vi "Armed Response.vi"(8 "error in (no error)":errorcluster, 9 "Armed":bool, 10 "Sender":string, 11 "Pulse Controller in":refnum<class "Pulse Controller.lvclass">) -> (0 "error out":errorcluster, 3 "Pulse Controller out":refnum<class "Pulse Controller.lvclass">)   [LabVIEW 2016, in "Pulse Controller.lvclass"]
uses:
  Pulse Controller.lvclass
  C:/github/LabActor/Controllers/Process Controller/Process Controller.lvclass
  C:/Program Files/National Instruments/LabVIEW 2016/vi.lib/ActorFramework/Actor/Actor.lvclass
  Process Controller/Process Controller.lvclass/Process Controller.ctl
  Pulse Controller.lvclass/Pulse Controller.ctl
  <vilib>/ActorFramework/Actor/Actor.lvclass/Actor.ctl
  Monitor-Pulse Messages/Update Armed Msg/Update Armed Msg.lvclass/Update Armed Msg.ctl
  <vilib>/ActorFramework/Message Enqueuer/Message Enqueuer.lvclass/Message Enqueuer.ctl
  Process Controller/Read Active measurements names.vi
  <vilib>/ActorFramework/Message Enqueuer/Enqueue.vi
  Monitor-Pulse Messages/Update Armed Msg/Update Armed Msg.lvclass
  C:/Program Files/National Instruments/LabVIEW 2016/vi.lib/ActorFramework/Message/Message.lvclass
  <vilib>/ActorFramework/Message Priority Queue/Priority Enqueue.vi
  <vilib>/ActorFramework/Actor/Actor.lvclass
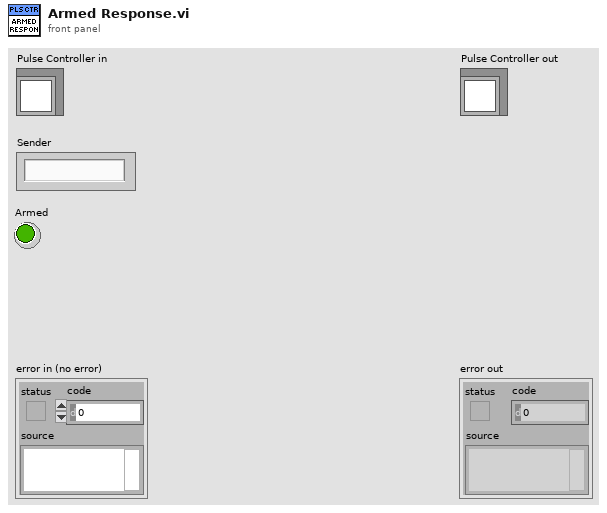
[diagram p1: front panel]
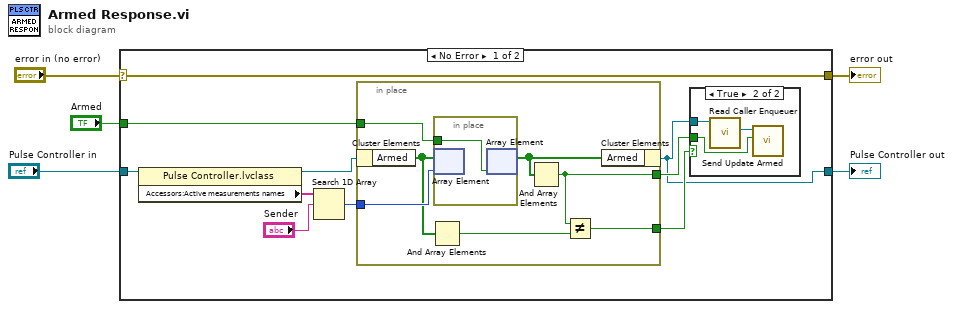
[diagram p0: block diagram]
diagram:
  n1 = case shown="No Error" "error in (no error)" {
    selector: "error in (no error)" -> [w14 w28]
    tunnel: [w14 w28] -> w4
    tunnel: [w6 w27] -> w2
    tunnel: "Pulse Controller in" -> [w15 w27]
    tunnel: "Armed" -> [w10 _]
    frame No Error {
      n2 = property class="Pulse Controller.lvclass"(reference=w15) -> (reference out=w9:refnum<class "Pulse Controller.lvclass">, "Accessors:Active measurements names"=w13:string[])  [unwired: 1 in, 1 out]
      n3 = Search 1D Array(1D array=w13, element="Sender") -> (index of element=w11:i32)  [unwired: 1 in]
      n4 = in-place {
        in-place-border: w11 -> [w25]
        in-place-border: w10 -> [w24]
        in-place-border: [w20] -> w8
        in-place-border: [w19] -> w7
        n5 = in-place-cluster #1(w9) -> ("Armed"=w23:bool[])
        n6 = And Array Elements(Boolean array=w23) -> (logical AND=w21:bool)
        n7 = in-place {
          in-place-border: w24 -> [w26]
          n8 = in-place-array #2(w23, w25) -> ()  [unwired: 1 out]
          n9 = in-place-array #2(w26) -> (w22:bool[])  [unwired: 1 out]
        }
        n10 = And Array Elements(Boolean array=w22) -> (logical AND=w19:bool)
        n11 = Not Equal?(x=w19, y=w21) -> (x != y?=w20:bool)
        n12 = in-place-cluster #1("Armed"=w22) -> (w6:refnum<class "Pulse Controller.lvclass">)
      }
      n13 = case shown="True" w8 {
        tunnel: w7 -> [_ w18]
        tunnel: w6 -> [_ w17]
        frame False {
        }
        frame True {
          n14 = call <vilib>:"Read Caller Enqueuer.vi"("Actor"=w17) -> ("Caller Enqueuer"=w16:refnum<class "Message Enqueuer.lvclass">)  [unwired: 10 in]
          n15 = call "Send Update Armed.vi"("Armed"=w18, "Message Enqueuer"=w16) -> ()  [unwired: 8 in, 2 out]
        }
      }
    }
    frame Error {
    }
  }
  "error out" <- w4
  "Pulse Controller out" <- w2
